vi "状态告警区.vi"(11 "数组":u16[](array[numeric]) format="%04xH") -> (3 "状态告警区":T1 {"工作状态" items=["空闲"=0, "水样测试"=1, "标样核查"=2, "零点核查"=3, "跨度核查"=4, "空白测试"=5, "平行样测试"=6, "加标回收"=7, "空白校准"=8, "标样校准"=9, "初始化（清洗）"=10, "调试"=22, "填充管路"=30, "清洗管路"=31, "清洗反应杯"=32]; "告警代码" items=["无告警", "缺试剂告警", "缺水样告警", "缺蒸馏水告警", "缺标液告警", "仪表漏液告警", "标定异常告警", "超量程告警", "加热异常", "低试剂预警", "超上限告警", "超下限告警", "仪表内部其他异常", "滴定异常告警", "电极异常告警", "量程切换告警", "参数设置告警", "PH电极电位异常", "电导率电极异常", "浊度光度异常", "溶解氧电极异常", "溶解氧光强异常", "温度异常告警", "PH异常告警", "溶解氧异常告警", "电导率异常告警", "浊度异常告警", "叶绿素异常告警", "藻密度异常告警", "蓝绿藻异常告警", "ORP异常告警", "氨氮异常告警", "清洁刷异常告警", "SD卡异常告警", "蓝牙异常告警", "Wifi异常告警", "流程异常告警"]; "故障代码" items=["无故障", "电机故障", "温度故障", "通讯故障", "滴定故障"]})   [LabVIEW 2016, in "斯坦道CODMn新电路板.lvlib"]
panel:
  # "共占用29 WORD"
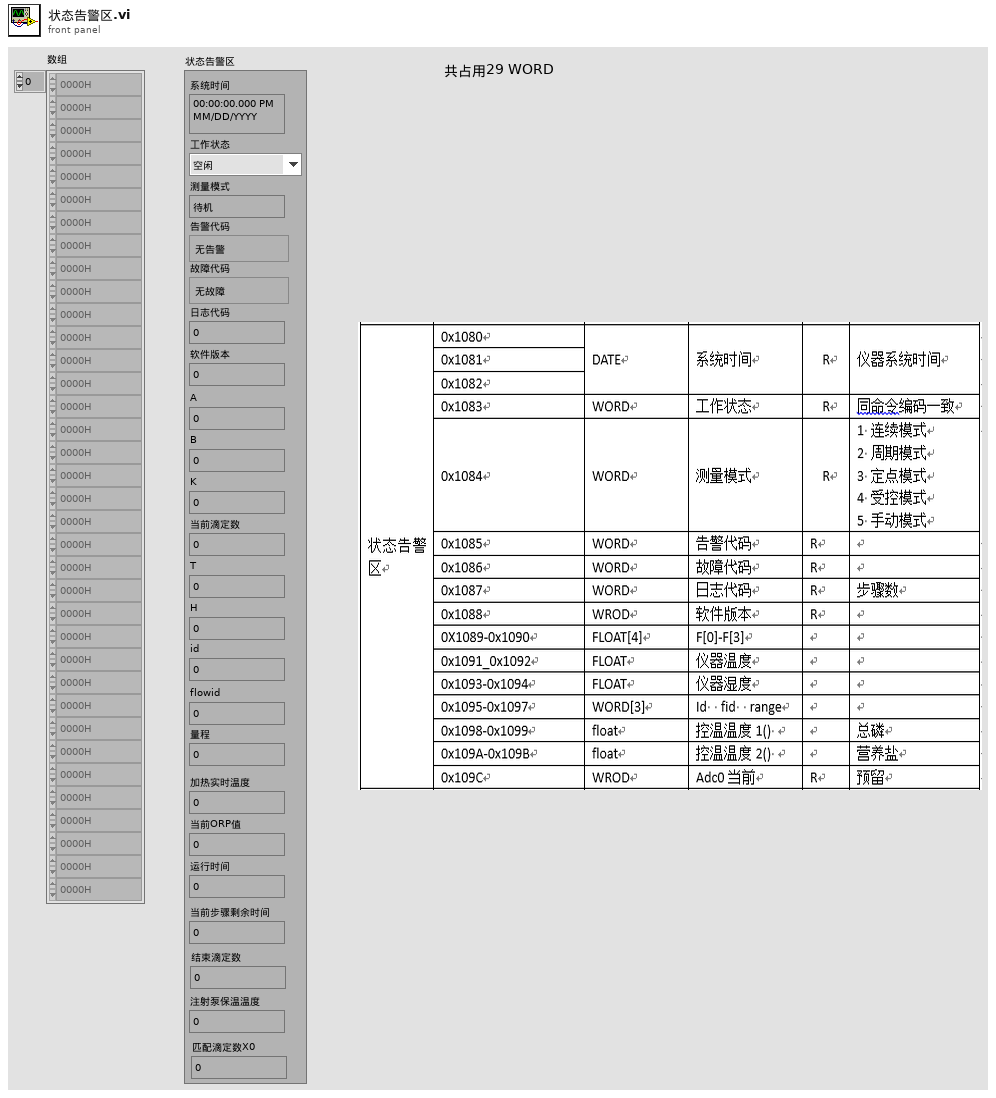
[diagram p1: front panel]
types:
  T1 = cluster{"系统时间":timestamp, "工作状态":u16, "测量模式":enum16{"待机", "连续模式", "周期模式", "定点模式", "受控模式", "手动模式"}, "告警代码":u16, "故障代码":u16, "日志代码":u16, "软件版本":u16, "A":sgl, "B":sgl, "K":sgl, "当前滴定数":sgl, "T":sgl, "H":sgl, "id":u16, "flowid":u16, "量程":u16, "加热实时温度":sgl, "当前ORP值":sgl, "运行时间":sgl, "当前步骤剩余时间":sgl, "结束滴定数":sgl, "注射泵保温温度":sgl, "匹配滴定数X0":u16}
  T2 = cluster{"time stamp":timestamp, "WORD":u16, "WORD":u16, "WORD":u16, "WORD":u16, "WORD":u16, "WORD":u16, "FLOAT":sgl, "FLOAT":sgl, "FLOAT":sgl, "FLOAT":sgl, "FLOAT":sgl, "FLOAT":sgl, "WORD":u16, "WORD":u16, "WORD":u16, "FLOAT":sgl, "FLOAT":sgl, "WORD":u16, "WORD":u16, "WORD":u16, "FLOAT":sgl, "WORD":u16}
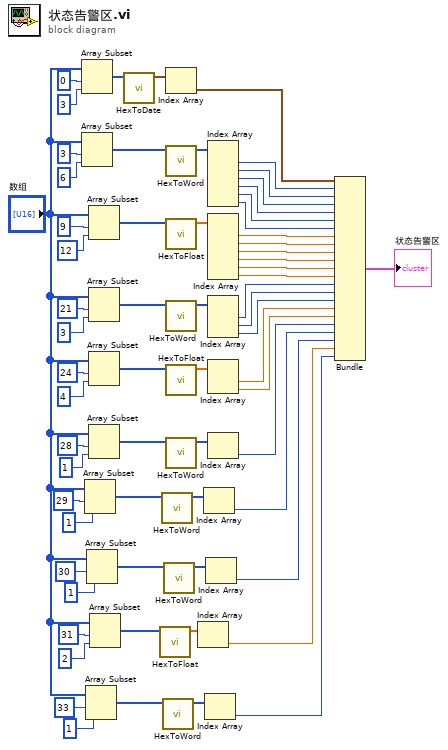
[diagram p0: block diagram]
diagram:
  n1 = Array Subset(array="数组", index=0 ("索引"), length=3 ("长度")) -> (w63:u16[])
  n2 = Array Subset(array="数组", index=3 ("索引"), length=6 ("长度")) -> (w58:u16[])
  n3 = Array Subset(array="数组", index=29 ("索引"), length=1 ("长度")) -> (w22:u16[])
  n4 = Array Subset(array="数组", index=33 ("索引"), length=1 ("长度")) -> (w5:u16[])
  n5 = Array Subset(array="数组", index=30 ("索引"), length=1 ("长度")) -> (w15:u16[])
  n6 = Array Subset(array="数组", index=9 ("索引"), length=12 ("长度")) -> (w48:u16[])
  n7 = Array Subset(array="数组", index=21 ("索引"), length=3 ("索引")) -> (w38:u16[])
  n8 = Array Subset(array="数组", index=24 ("索引"), length=4 ("索引")) -> (w31:u16[])
  n9 = Array Subset(array="数组", index=28 ("索引"), length=1 ("长度")) -> (w26:u16[])
  n10 = Array Subset(array="数组", index=31 ("索引"), length=2 ("索引")) -> (w10:u16[])
  n11 = call "HexToDate.vi"("数组"=w63) -> ("DATE"=w60:timestamp[])  [unwired: 10 in]
  n12 = call "HexToFloat.vi"("数组"=w10) -> ("FLOAT"=w9:sgl[])  [unwired: 10 in]
  n13 = call "HexToWord.vi"("数组"=w22) -> ("WORD"=w21:u16[])  [unwired: 10 in]
  n14 = call "HexToWord.vi"("数组"=w5) -> ("WORD"=w4:u16[])  [unwired: 10 in]
  n15 = call "HexToWord.vi"("数组"=w15) -> ("WORD"=w16:u16[])  [unwired: 10 in]
  n16 = Index Array(array=w60) -> (element=w59:timestamp)  [unwired: 1 in]
  n17 = call "HexToWord.vi"("数组"=w58) -> ("WORD"=w57:u16[])  [unwired: 10 in]
  n18 = call "HexToFloat.vi"("数组"=w48) -> ("FLOAT"=w47:sgl[])  [unwired: 10 in]
  n19 = call "HexToWord.vi"("数组"=w38) -> ("WORD"=w37:u16[])  [unwired: 10 in]
  n20 = call "HexToFloat.vi"("数组"=w31) -> ("FLOAT"=w30:sgl[])  [unwired: 10 in]
  n21 = call "HexToWord.vi"("数组"=w26) -> ("WORD"=w27:u16[])  [unwired: 10 in]
  n22 = Index Array(array=w9) -> (element=w7:sgl)  [unwired: 1 in]
  n23 = Index Array(array=w21) -> (element=w20:u16)  [unwired: 1 in]
  n24 = Index Array(array=w4) -> (element=w1:u16)  [unwired: 1 in]
  n25 = Index Array(array=w16) -> (element=w13:u16)  [unwired: 1 in]
  n26 = Index Array(array=w57) -> (element #1=w56:u16, element #2=w55:u16, element #3=w54:u16, element #4=w53:u16, element #5=w52:u16, element #6=w51:u16)  [unwired: 6 in]
  n27 = Index Array(array=w47) -> (element #1=w46:sgl, element #2=w45:sgl, element #3=w44:sgl, element #4=w43:sgl, element #5=w42:sgl, element #6=w41:sgl)  [unwired: 6 in]
  n28 = Index Array(array=w37) -> (element #1=w36:u16, element #2=w35:u16, element #3=w34:u16)  [unwired: 3 in]
  n29 = Index Array(array=w30) -> (element #1=w29:sgl, element #2=w28:sgl)  [unwired: 2 in]
  n30 = Index Array(array=w27) -> (element=w24:u16)  [unwired: 1 in]
  n31 = Bundle("time stamp"=w59, "WORD"=w56, "WORD"=w55, "WORD"=w54, "WORD"=w53, "WORD"=w52, "WORD"=w51, "FLOAT"=w46, "FLOAT"=w45, "FLOAT"=w44, "FLOAT"=w43, "FLOAT"=w42, "FLOAT"=w41, "WORD"=w36, "WORD"=w35, "WORD"=w34, "FLOAT"=w29, "FLOAT"=w28, "WORD"=w24, "WORD"=w20, "WORD"=w13, "FLOAT"=w7, "WORD"=w1) -> (→"状态告警区":T2)  [unwired: 1 in]
